vi "WriteDeviceModel.vi"(8 "error in (no error)":errorcluster, 11 "device model":T1) -> (0 "error out":errorcluster)   [LabVIEW 2017, in "ServerComm.lvlib"]
uses:
  <vilib>/addons/InsightCM/Devices/Shared/Common/ServerComm/ServerComm.lvlib
  <vilib>/addons/InsightCM/MessageBus/Base/controls/R2_DeviceModel.ctl
  <vilib>/addons/InsightCM/MessageBus/Base/controls/R2_Device.ctl
  <vilib>/addons/InsightCM/MessageBus/Base/controls/KeyValuePair.ctl
  <vilib>/addons/InsightCM/MessageBus/Base/controls/DeviceState.ctl
  <vilib>/addons/InsightCM/MessageBus/Base/controls/R2_DataGroup.ctl
  <vilib>/addons/InsightCM/MessageBus/Base/controls/OperatingState.ctl
  <vilib>/addons/InsightCM/MessageBus/Base/controls/Trigger.ctl
  <vilib>/addons/InsightCM/MessageBus/Base/controls/Condition.ctl
  <vilib>/addons/InsightCM/MessageBus/Base/controls/BurstModeTrigger.ctl
  <vilib>/addons/InsightCM/MessageBus/Base/controls/SensorGroup.ctl
  <vilib>/addons/InsightCM/MessageBus/Base/controls/Endpoint.ctl
  <vilib>/addons/InsightCM/MessageBus/Base/controls/WirelessChannel.ctl
  <vilib>/addons/InsightCM/MessageBus/Base/controls/R2_Channel.ctl
  <vilib>/addons/InsightCM/MessageBus/Base/controls/Metric.ctl
  <vilib>/addons/InsightCM/MessageBus/Base/controls/Tag.ctl
  <vilib>/addons/InsightCM/Utilities/GlobalConfiguration/GlobalConfiguration.lvlib
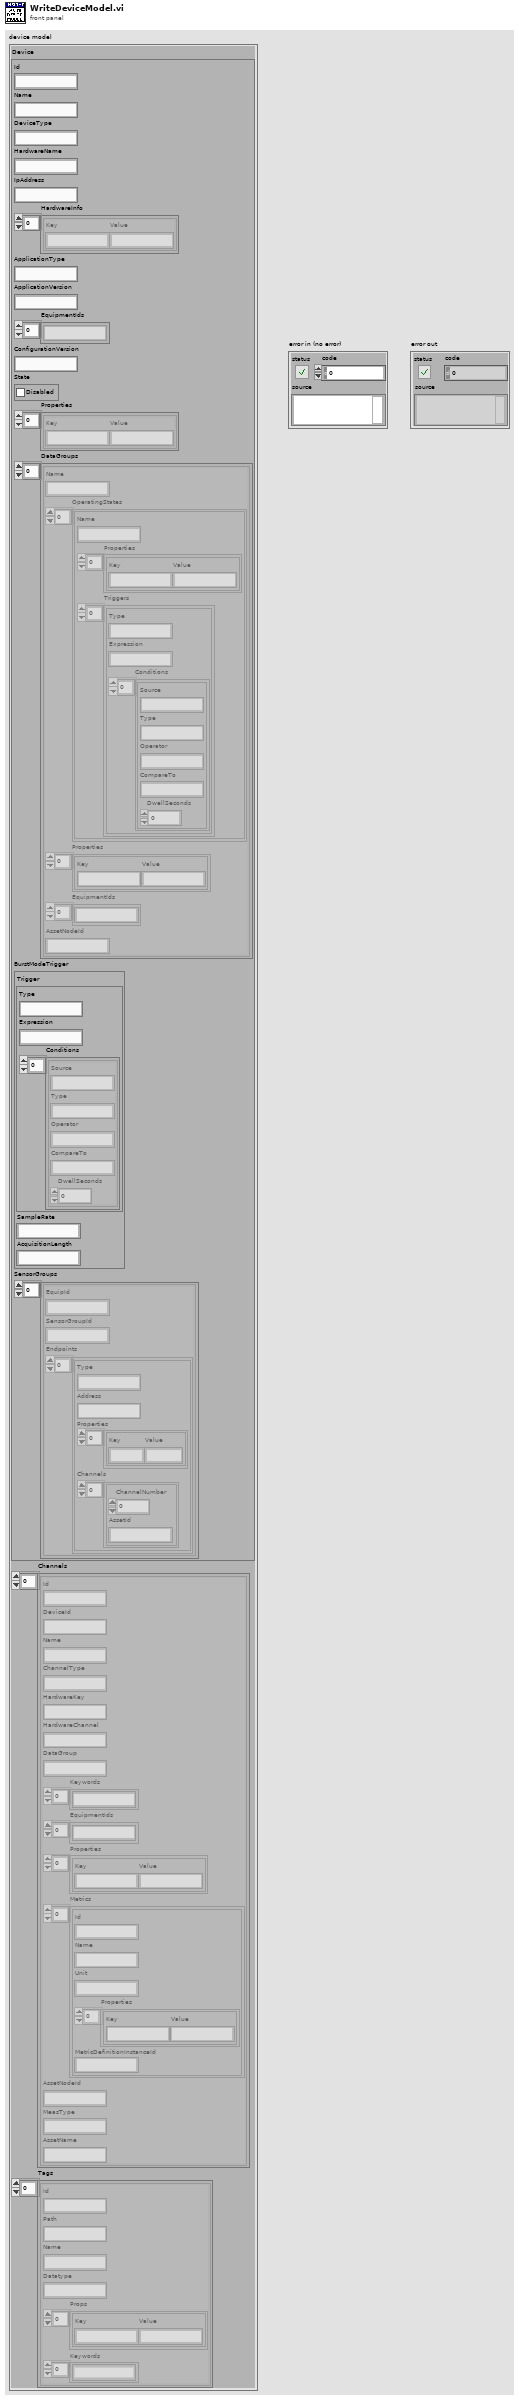
[diagram p1: front panel]
types:
  T1 = typedef "R2_DeviceModel.ctl" = cluster{"Device":T2, "Channels":T13[], "Tags":T15[]}
  T2 = typedef "R2_Device.ctl" = cluster{"Id":string, "Name":string, "DeviceType":string, "HardwareName":string, "IpAddress":string, "HardwareInfo":T3[], "ApplicationType":string, "ApplicationVersion":string, "EquipmentIds":string[], "ConfigurationVersion":string, "State":T4, "Properties":T3[], "DataGroups":T5[], "BurstModeTrigger":T9, "SensorGroups":T10[]}
  T3 = typedef "KeyValuePair.ctl" = cluster{"Key":string, "Value":string}
  T4 = typedef "DeviceState.ctl" = cluster{"Disabled":bool}
  T5 = typedef "R2_DataGroup.ctl" = cluster{"Name":string, "OperatingStates":T6[], "Properties":T3[], "EquipmentIds":string[], "AssetNodeId":string}
  T6 = typedef "OperatingState.ctl" = cluster{"Name":string, "Properties":T3[], "Triggers":T7[]}
  T7 = typedef "Trigger.ctl" = cluster{"Type":string, "Expression":string, "Conditions":T8[]}
  T8 = typedef "Condition.ctl" = cluster{"Source":string, "Type":string, "Operator":string, "CompareTo":string, "DwellSeconds":dbl}
  T9 = typedef "BurstModeTrigger.ctl" = cluster{"Trigger":T7, "SampleRate":string, "AcquisitionLength":string}
  T10 = typedef "SensorGroup.ctl" = cluster{"EquipId":string, "SensorGroupId":string, "Endpoints":T11[]}
  T11 = typedef "Endpoint.ctl" = cluster{"Type":string, "Address":string, "Properties":T3[], "Channels":T12[]}
  T12 = typedef "WirelessChannel.ctl" = cluster{"ChannelNumber":i32, "AssetId":string}
  T13 = typedef "R2_Channel.ctl" = cluster{"Id":string, "DeviceId":string, "Name":string, "ChannelType":string, "HardwareKey":string, "HardwareChannel":string, "DataGroup":string, "Keywords":string[], "EquipmentIds":string[], "Properties":T3[], "Metrics":T14[], "AssetNodeId":string, "MeasType":string, "AssetName":string}
  T14 = typedef "Metric.ctl" = cluster{"Id":string, "Name":string, "Unit":string, "Properties":T3[], "MetricDefinitionInstanceId":string}
  T15 = typedef "Tag.ctl" = cluster{"Id":string, "Path":string, "Name":string, "Datatype":string, "Props":T3[], "Keywords":string[]}
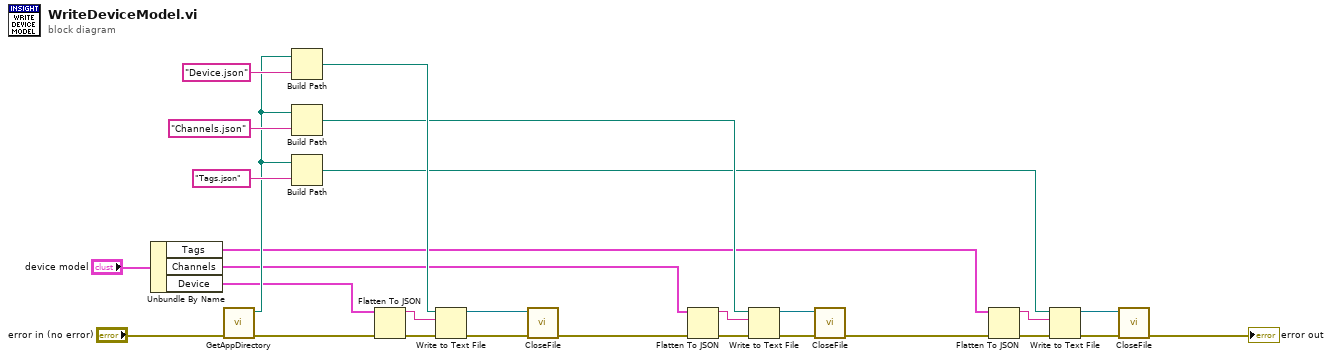
[diagram p0: block diagram]
diagram:
  n1 = Unbundle By Name("device model") -> ("Tags"=w10:T15[], "Channels"=w11:T13[], "Device"=w12:T2)
  n2 = call <vilib>:"GetAppDirectory.vi"("error in (no error)"="error in (no error)") -> ("error out"=w26:errorcluster, "application directory"=w21:path)  [unwired: 9 in]
  n3 = Build Path(base path=w21, name or relative path="Device.json") -> (appended path=w20:path)
  n4 = Build Path(base path=w21, name or relative path="Channels.json") -> (appended path=w15:path)
  n5 = Build Path(base path=w21, name or relative path="Tags.json") -> (appended path=w14:path)
  n6 = Flatten To JSON(anything=w12, error in (no error)=w26) -> (JSON string=w24:string, 11:w25:errorcluster)  [unwired: 1 in]
  n7 = Write to Text File(file (use dialog)=w20, text=w24, error in=w25) -> (refnum out=w9:refnum<file>, error out=w8:errorcluster)  [unwired: 1 in, 1 out]
  n8 = call <vilib>:"CloseFile.vi"("error in (no error)"=w8, "file reference"=w9) -> ("error out"=w7:errorcluster)  [unwired: 9 in]
  n9 = Flatten To JSON(anything=w11, error in (no error)=w7) -> (JSON string=w19:string, 11:w18:errorcluster)  [unwired: 1 in]
  n10 = Write to Text File(file (use dialog)=w15, text=w19, error in=w18) -> (refnum out=w6:refnum<file>, error out=w5:errorcluster)  [unwired: 1 in, 1 out]
  n11 = call <vilib>:"CloseFile.vi"("error in (no error)"=w5, "file reference"=w6) -> ("error out"=w4:errorcluster)  [unwired: 9 in]
  n12 = Flatten To JSON(anything=w10, error in (no error)=w4) -> (JSON string=w16:string, 11:w17:errorcluster)  [unwired: 1 in]
  n13 = Write to Text File(file (use dialog)=w14, text=w16, error in=w17) -> (refnum out=w3:refnum<file>, error out=w2:errorcluster)  [unwired: 1 in, 1 out]
  n14 = call <vilib>:"CloseFile.vi"("error in (no error)"=w2, "file reference"=w3) -> ("error out"=→"error out":errorcluster)  [unwired: 9 in]
